vi "GOOP_DrawWirePreview_Simple.vi"(10 "WireLength(X)":i16=100, 11 "WireConfiguration":T1={"Edge thickness"=1, "Edge color"=6916708, "Center thickness"=1, "Center pattern"=enum."Solid", "CenterColor1"=8882055, "CenterColor2"=0, "Tunnels and terminals colors"=16711680}) -> (3 "WirePicture":picture)   [LabVIEW 2020]
uses:
  <resource>/Framework/Providers/Open_GDS/SubVIs/GOOP_WireConfigurationType.ctl
  <resource>/Framework/Providers/Open_GDS/SubVIs/GOOP_WirePattern.ctl
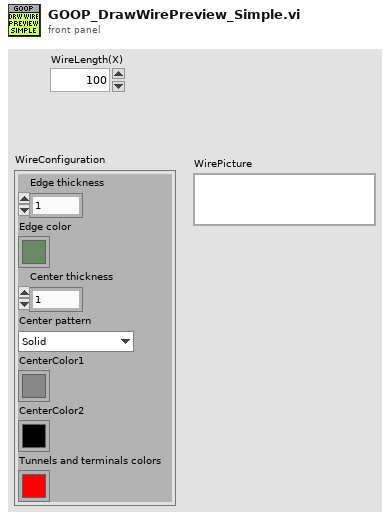
[diagram p1: front panel]
types:
  T1 = typedef "GOOP_WireConfigurationType.ctl" = cluster{"Edge thickness":i32, "Edge color":u32, "Center thickness":i32, "Center pattern":T2, "CenterColor1":u32, "CenterColor2":u32, "Tunnels and terminals colors":u32}
  T2 = typedef "GOOP_WirePattern.ctl" = enum16{"Solid", "Large dash", "Small dash"}
  T3 = typedef "imagedata.ctl" = cluster{"image type":i32, "image depth":i32, "image":u8[], "mask":u8[], "colors":u32[], "Rectangle":cluster{"left":i16, "top":i16, "right":i16, "bottom":i16}}
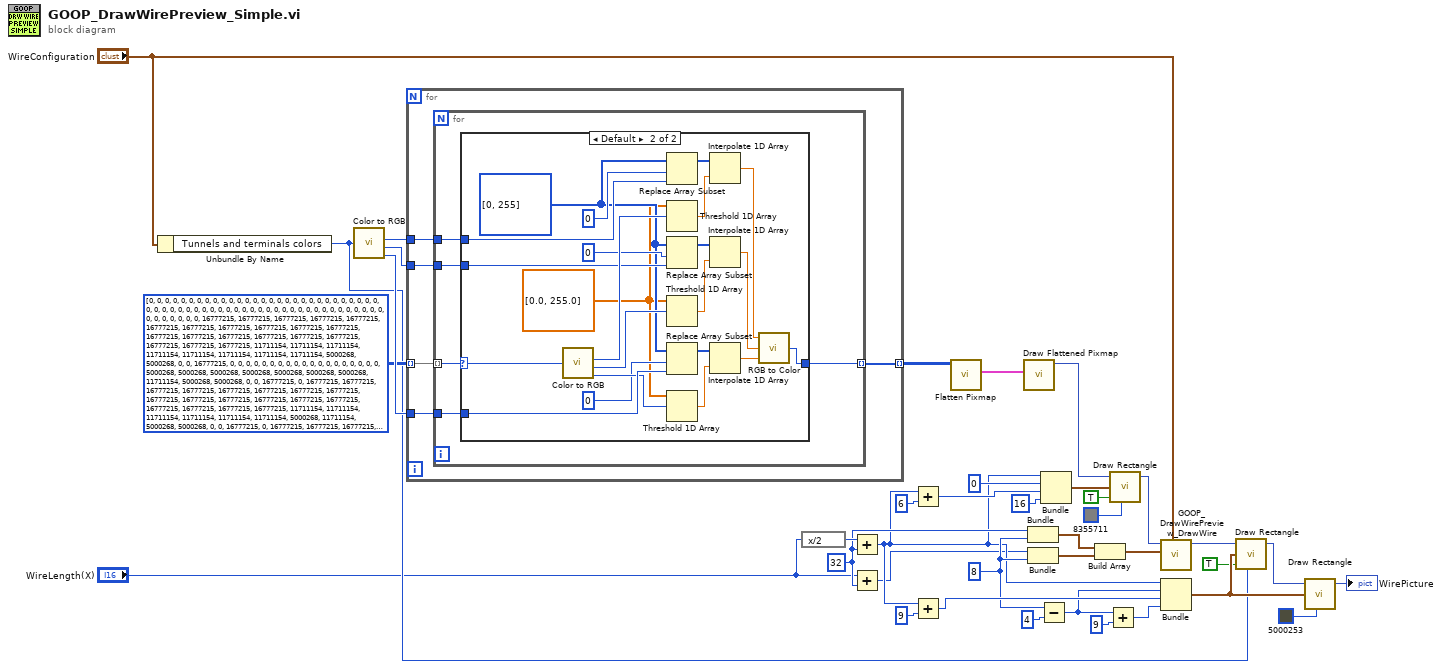
[diagram p0: block diagram]
diagram:
  w16 = i16 8 ("y")
  w4 = i16 32 ("x")
  n1 = Unbundle By Name("WireConfiguration") -> ("Tunnels and terminals colors"=w6:u32)
  n2 = call <vilib>:"Color to RGB.vi"("Color"=w6) -> ("R"=w37:u8, "G"=w36:u8, "B"=w35:u8)  [unwired: 1 out]
  n3 = for {
    tunnel: u32[][] [[0, 0, 0, 0, 0, 0, 0, 0, 0, 0, 0, 0, 0, 0, 0, 0, 0, 0, 0, 0, 0, 0, 0, 0, 0, 0, 0, 0, 0, 0, 0, 0], [0, 0, 0, 0, 0, 0, 0, 0, 0, 0, 0, 0, 0, 0, 0, 0, 0, 0, 0, 0, 0, 0, 0, 0, 0, 0, 0, 0, 0, 0, 0, 0], [0, 0, 16777215, 16777215, 16777215, 16777215, 16777215, 16777215, 16777215, 16777215, 16777215, 16777215, 16777215, 16777215, 16777215, 16777215, 16777215, 16777215, 16777215, 16777215, 16777215, 16777215, 11711154, 11711154, 11711154, 11711154, 11711154, 11711154, 11711154, 11711154, 5000268, 5000268], [0, 0, 16777215, 0, 0, 0, 0, 0, 0, 0, 0, 0, 0, 0, 0, 0, 0, 0, 0, 0, 0, 0, 5000268, 5000268, 5000268, 5000268, 5000268, 5000268, 5000268, 11711154, 5000268, 5000268], [0, 0, 16777215, 0, 16777215, 16777215, 16777215, 16777215, 16777215, 16777215, 16777215, 16777215, 16777215, 16777215, 16777215, 16777215, 16777215, 16777215, 16777215, 16777215, 16777215, 16777215, 11711154, 11711154, 11711154, 11711154, 11711154, 11711154, 5000268, 11711154, 5000268, 5000268], [0, 0, 16777215, 0, 16777215, 16777215, 16777215, 16777215, 16777215, 0, 0, 0, 16777215, 16777215, 0, 0, 0, 0, 16777215, 16777215, 16777215, 16777215, 5000268, 5000268, 11711154, 11711154, 11711154, 0, 5000268, 11711154, 5000268, 5000268], [0, 0, 16777215, 0, 16777215, 16777215, 16777215, 16777215, 0, 0, 16777215, 0, 0, 16777215, 0, 0, 16777215, 0, 0, 16777215, 16777215, 16777215, 5000268, 5000268, 11711154, 11711154, 11711154, 0, 0, 11711154, 5000268, 5000268], [0, 0, 16777215, 0, 16777215, 16777215, 16777215, 16777215, 0, 0, 16777215, 0, 0, 16777215, 0, 0, 0, 0, 16777215, 16777215, 16777215, 16777215, 5000268, 5000268, 11711154, 11711154, 11711154, 0, 0, 0, 5000268, 5000268], [0, 0, 16777215, 0, 16777215, 16777215, 16777215, 16777215, 0, 0, 16777215, 0, 0, 16777215, 0, 0, 16777215, 0, 0, 16777215, 0, 16777215, 5000268, 5000268, 11711154, 11711154, 11711154, 0, 0, 0, 5000268, 5000268], [0, 0, 16777215, 0, 16777215, 16777215, 16777215, 16777215, 0, 0, 16777215, 0, 0, 16777215, 0, 0, 16777215, 0, 0, 16777215, 0, 16777215, 5000268, 5000268, 11711154, 11711154, 11711154, 0, 0, 11711154, 5000268, 5000268], [0, 0, 16777215, 0, 16777215, 16777215, 16777215, 16777215, 16777215, 0, 0, 0, 16777215, 16777215, 0, 0, 0, 0, 16777215, 16777215, 16777215, 0, 5000268, 11711154, 11711154, 11711154, 11711154, 0, 5000268, 11711154, 5000268, 5000268], [0, 0, 16777215, 0, 16777215, 16777215, 16777215, 16777215, 16777215, 16777215, 16777215, 16777215, 16777215, 16777215, 16777215, 16777215, 16777215, 16777215, 16777215, 16777215, 16777215, 16777215, 11711154, 11711154, 11711154, 11711154, 11711154, 11711154, 5000268, 11711154, 5000268, 5000268], [0, 0, 16777215, 0, 0, 0, 0, 0, 0, 0, 0, 0, 0, 0, 0, 0, 0, 0, 0, 0, 0, 0, 5000268, 5000268, 5000268, 5000268, 5000268, 5000268, 5000268, 11711154, 5000268, 5000268], [0, 0, 16777215, 16777215, 16777215, 16777215, 16777215, 16777215, 16777215, 16777215, 16777215, 16777215, 16777215, 16777215, 16777215, 16777215, 16777215, 16777215, 16777215, 16777215, 16777215, 16777215, 11711154, 11711154, 11711154, 11711154, 11711154, 11711154, 11711154, 11711154, 5000268, 5000268], [0, 0, 0, 0, 0, 0, 0, 0, 0, 0, 0, 0, 0, 0, 0, 0, 0, 0, 0, 0, 0, 0, 0, 0, 0, 0, 0, 0, 0, 0, 0, 0], [0, 0, 0, 0, 0, 0, 0, 0, 0, 0, 0, 0, 0, 0, 0, 0, 0, 0, 0, 0, 0, 0, 0, 0, 0, 0, 0, 0, 0, 0, 0, 0]] ("24-bit pixmap") -> [w43] mode=indexing
    tunnel: w37 -> [w42]
    tunnel: w36 -> [w41]
    tunnel: w35 -> [w40]
    tunnel: [w39] -> w34 mode=indexing
    n4 = for {
      tunnel: w43 -> [w48] mode=indexing
      tunnel: w42 -> [w47]
      tunnel: w41 -> [w44]
      tunnel: w40 -> [w46]
      tunnel: [w45] -> w39 mode=indexing
      n5 = case shown="Default" w48 {
        selector: w48 -> [w49 w71]
        tunnel: w47 -> [_ w70]
        tunnel: w46 -> [_ w69]
        tunnel: [w49 w68] -> w45
        tunnel: w44 -> [_ w64]
        frame 16777215 {
        }
        frame Default {
          w53 = u8[] [0, 255]
          w52 = sgl[] [0.0, 255.0]
          n6 = call <vilib>:"Color to RGB.vi"("Color"=w71) -> ("R"=w67:u8, "G"=w66:u8, "B"=w65:u8)  [unwired: 1 out]
          n7 = Replace Array Subset(array=w53, new element=w70, index=0) -> (w62:u8[])
          n8 = Threshold 1D Array(2:w67, 3:w52) -> (0:w56:sgl)  [unwired: 1 in]
          n9 = Replace Array Subset(array=w53, new element=w64, index=0) -> (w60:u8[])
          n10 = Threshold 1D Array(2:w66, 3:w52) -> (0:w51:sgl)  [unwired: 1 in]
          n11 = Replace Array Subset(array=w53, new element=w69, index=0) -> (w57:u8[])
          n12 = Threshold 1D Array(2:w65, 3:w52) -> (0:w50:sgl)  [unwired: 1 in]
          n13 = Interpolate 1D Array(1:w56, 2:w62) -> (0:w61:dbl)
          n14 = Interpolate 1D Array(1:w51, 2:w60) -> (0:w55:dbl)
          n15 = Interpolate 1D Array(1:w50, 2:w57) -> (0:w54:dbl)
          n16 = call <vilib>:"RGB to Color.vi"("B"=w54, "G"=w55, "R"=w61) -> ("Color"=w68:u32)
        }
      }
    }
  }
  n17 = expression code="x/2"("WireLength(X)") -> (w5:i16)
  n18 = Add(x=w5, y=w4) -> (x+y=w3:i16)
  n19 = Add(x="WireLength(X)", y=w4) -> (x+y=w1:i16)
  n20 = Add(x=w3, y=i16 6) -> (x+y=w28:i16)
  n21 = Add(x=w3, y=i16 9) -> (x+y=w21:i16)
  n22 = call <vilib>:"Flatten Pixmap.vi"("24-bit pixmap"=w34) -> ("image data"=w38:T3)  [unwired: 10 in]
  n23 = call <vilib>:"Draw Flattened Pixmap.vi"("image data"=w38) -> ("new picture"=w31:picture)  [unwired: 8 in]
  n24 = Bundle("x"=w4, "y"=w16) -> (w19:cluster{"x":i16, "y":i16})  [unwired: 1 in]
  n25 = Bundle(w1, "y"=w16) -> (w18:cluster{i16, "y":i16})  [unwired: 1 in]
  n26 = Subtract(x=w16, y=i16 4) -> (x-y=w14:i16)
  n27 = Bundle(w3, "index"=i16 0, w28, "index"=i16 16) -> (w23:cluster{i16, "index":i16, i16, "index":i16})  [unwired: 1 in]
  n28 = Build Array(w19, w18) -> (w17:cluster{"x":i16, "y":i16}[])
  n29 = Add(x=w14, y=i16 9) -> (x+y=w12:i16)
  n30 = call <vilib>:"Draw Rectangle.vi"("picture"=w31, "rect"=w23, "fill?(F)"=TRUE, "color(black)"=u32 8355711) -> ("new picture"=w30:picture)  [unwired: 5 in]
  n31 = call <resource>:"GOOP_DrawWirePreview_DrawWire.vi"("WireConfiguration"="WireConfiguration", "Array"=w17, "PictureIn"=w30) -> ("PictureOut"=w10:picture)  [unwired: 8 in]
  n32 = Bundle(w3, w14, w21, w12) -> (w8:cluster{i16, i16, i16, i16})  [unwired: 1 in]
  n33 = call <vilib>:"Draw Rectangle.vi"("picture"=w10, "rect"=w8, "fill?(F)"=TRUE, "color(black)"=w6) -> ("new picture"=w9:picture)  [unwired: 5 in]
  n34 = call <vilib>:"Draw Rectangle.vi"("picture"=w9, "rect"=w8, "color(black)"=u32 5000253) -> ("new picture"=→"WirePicture":picture)  [unwired: 6 in]
